vi "subset.vi"(1 "subset length":i32(slide)=307 scale=0.0..800.0, 2 "Index":i32, 3 "in array":dbl[](array[numeric])) -> (0 "subarray":dbl[](array[numeric]))   [LabVIEW 2009]
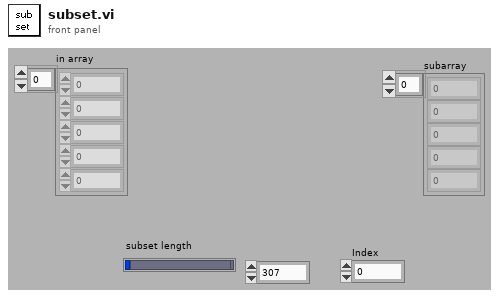
[diagram p1: front panel]
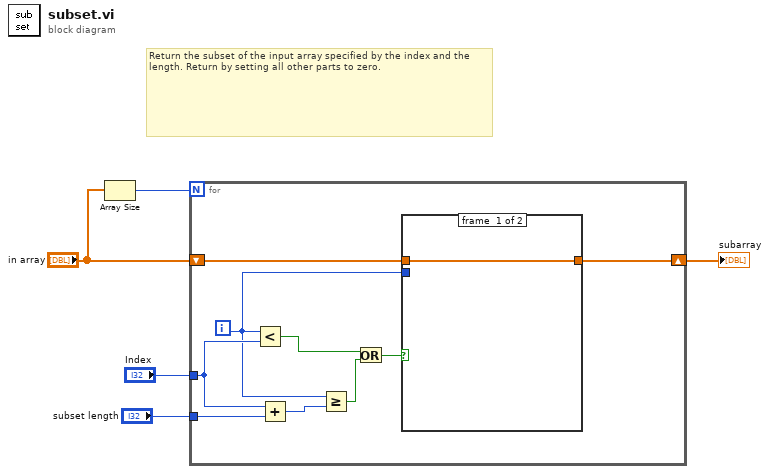
[diagram p0: block diagram]
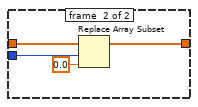
[diagram p2: hidden frame]
diagram:
  # "Return the subset of the input array specified by the index and the length. Return by setting all other parts to zero."
  n1 = Array Size(array="in array") -> (size(s)=w1:i32)
  n2 = for {
    N: w1 -> [_]
    tunnel: "Index" -> [w13]
    shift-right: [w6] -> w2
    shift-left: "in array" -> [w9]
    tunnel: "subset length" -> [w12]
    i -> [w7]
    n3 = Less?(x=w7, y=w13) -> (x < y?=w14:bool)
    n4 = Add(x=w13, y=w12) -> (x+y=w11:i32)
    n5 = Greater Or Equal?(x=w7, y=w11) -> (x >= y?=w10:bool)
    n6 = Or(x=w14, y=w10) -> (x .or. y?=w8:bool)
    n7 = case shown="False" w8 {
      tunnel: w9 -> [w15 w19]
      tunnel: w7 -> [_ w17]
      tunnel: [w15 w16] -> w6
      frame #0 {
      }
      frame #1 {
        n8 = Replace Array Subset(array=w19, new element=0.0 ("new element/subarray"), index=w17) -> (w16:dbl[])
      }
    }
  }
  "subarray" <- w2
